vi "Lab 2 Part B.vi"() -> ()   [LabVIEW 2020]
uses:
  <vilib>/MakerHub/LINX/Public/Utilities/Open Serial.vi
  <vilib>/addons/control/pid/pid.llb/PID (DBL).vi
  <vilib>/MakerHub/LINX/LMH-LINX.lvlib
  <vilib>/addons/control/pid/NI_PID_pid.lvlib
panel:
  in  "Amplitude":dbl=0.5
  in  "Frequency":dbl=0.01
  in  "Offset":dbl=1.5
  in  "PWM Channel":u8=10
  in  "AI1 and AI2 Channels":u8[](array[numeric])
  in  "Hall Channel":u8
  in  "Stop Button":bool
  out "Voltage":dbl
  in  "PID gains":T1={"proportional gain (Kc)"=5.0, "integral time (Ti, min)"=0.003, "derivative time (Td, min)"=0.01} {"derivative time (Td, min)" format="%.6f"; "integral time (Ti, min)" format="%.6f"; "proportional gain (Kc)" format="%.3f"}
  out "Output Chart":dynamicdata(graph)
  in  "output range":cluster{"output high":dbl, "output low":dbl}={"output high"=100.0, "output low"=-100.0} {"output low" format="%.2f"; "output high" format="%.2f"}
  out "Duty Cycle":dbl
  in  "Serial Port":refnum<visa-resource-name>="N/A"
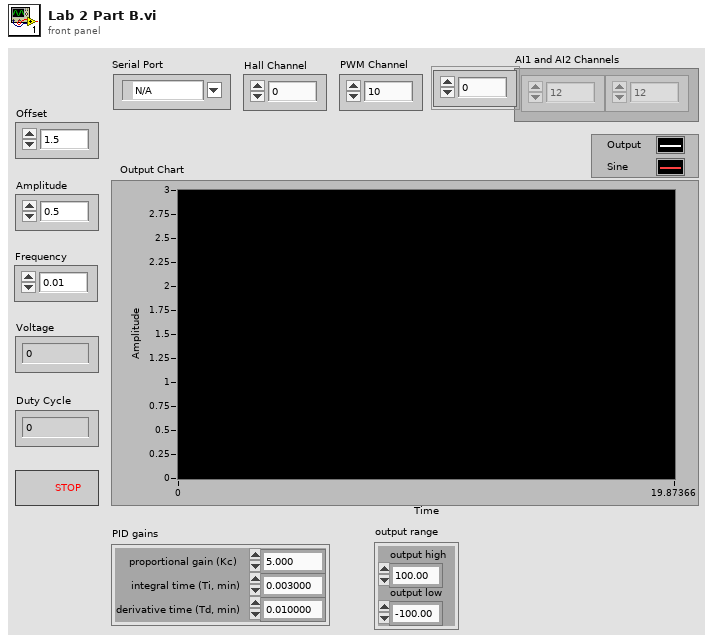
[diagram p1: front panel]
types:
  T1 = cluster{"proportional gain (Kc)":dbl, "integral time (Ti, min)":dbl, "derivative time (Td, min)":dbl}
  T2 = typedef "LMH-LINX.lvlib/LINX Ref.ctl" = cluster{"IO":T3, "Interface":T4, "LINX Device Config":T5}
  T3 = typedef "LMH-LINX.lvlib/Platform.ctl" = enum16{"Remote", "Local"}
  T4 = typedef "LMH-LINX.lvlib/Interface.ctl" = enum16{"Serial", "TCP"}
  T5 = typedef "LMH-LINX.lvlib/Device.lvlib/LINX Device Config.ctl" = cluster{"Interface":T4, "COM Port":refnum<visa-resource-name>, "TCP Configuration":T6, "Device Family":u8, "Device ID":u8, "Device Name":string, "TCP Ref":refnum<k5>, "Channels":T7}
  T6 = typedef "LMH-LINX.lvlib/Device.lvlib/TCP Config.ctl" = cluster{"IP Address":string, "Port":u16}
  T7 = typedef "LMH-LINX.lvlib/Channels.ctl" = cluster{"DI":u8[], "DO":u8[], "AI":u8[], "AO":u8[], "PWM":u8[], "QE":u8[], "UART":u8[], "I2C 2":u8[], "SPI":u8[], "CAN":u8[], "Servo":u8[], "AI Ref (V)":dbl, "AI Resolution (Bits)":u8, "AO Ref (V)":dbl, "AO Resolution (Bits)":u8}
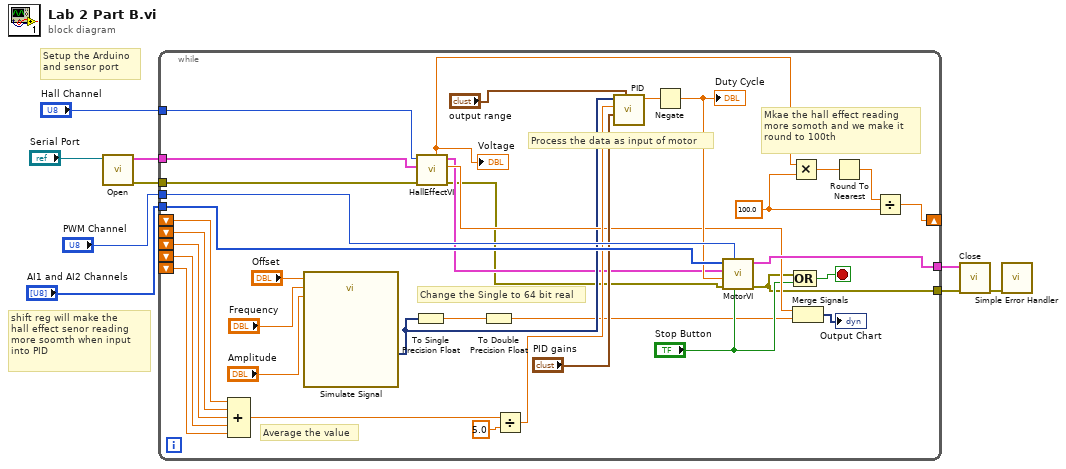
[diagram p0: block diagram]
diagram:
  # "shift reg will make the\nhall effect senor reading\nmore soomth when input \ninto PID"
  # "Setup the Arduino\nand sensor port"
  n1 = call-poly <vilib>:"Open.vi"("Serial Port"="Serial Port") -> ("Error Out"=w4:errorcluster, "LINX Resource"=w5:T2)  [unwired: 8 in, 1 out]
  n2 = while {
    tunnel: "Hall Channel" -> [w45]
    tunnel: "AI1 and AI2 Channels" -> [w44]
    tunnel: "PWM Channel" -> [w43]
    tunnel: w5 -> [w42]
    tunnel: w4 -> [w38]
    tunnel: [w39] -> w3
    tunnel: [w10] -> w2
    shift-right: [w23] -> _
    shift-left: _ -> [w36]
    shift-left: _ -> [w35]
    shift-left: _ -> [w34]
    shift-left: _ -> [w33]
    shift-left: _ -> [w29]
    stop <- w37 stop-if-true
    w24 = 100.0 ("y")
    # "Change the Single to 64 bit real"
    # "Average the value"
    # "Process the data as input of motor"
    # "Mkae the hall effect reading\nmore somoth and we make it\nround to 100th"
    n3 = Compound Arithmetic op=ADD(w36, w35, w34, w33, w29) -> (w32:dbl)
    n4 = call "Simulate Signal"("Offset"="Offset", "Frequency"="Frequency", "Amplitude"="Amplitude") -> ("Sine"=w16:dynamicdata)  [unwired: 11 in, 1 out]
    n5 = To Single Precision Float(number=w16) -> (single precision float=w13:sgl)
    n6 = call "HallEffectVI.vi"("error in (no error)"=w38, "LINX Resource in"=w42, "Analog Channel"=w45) -> ("error out"=w11:errorcluster, "Waveform Chart"=w22:dbl, "LINX Resource out"=w12:T2, "Voltage"=w27:dbl)  [unwired: 5 in]
    "Voltage" <- w27
    n7 = To Double Precision Float(number=w13) -> (double precision float=w14:dbl)
    n8 = Divide(x=w32, y=5.0) -> (x/y=w28:dbl)
    n9 = call-poly <vilib>:"PID.vi"("output range"="output range", "PID gains"="PID gains", "process variable"=w28, "setpoint"=w16) -> ("output"=w17:dbl)  [unwired: 6 in, 1 out]
    n10 = Negate(x=w17) -> (-x=w30:dbl)
    "Duty Cycle" <- w30
    n11 = call "MotorVI.vi"("stop"="Stop Button", "PWM Channel"=w43, "error in (no error)"=w11, "Duty Cycle (-100 to +100)"=w30, "LINX Resource in"=w12, "AI1 and AI2 Channels"=w44) -> ("error out"=w10:errorcluster, "LINX Resource out"=w39:T2)  [unwired: 3 in, 1 out]
    n12 = Multiply(x=w27, y=w24) -> (x*y=w26:dbl)
    n13 = Merge Signals(w22, w14) -> (→"Output Chart":dynamicdata)
    n14 = Compound Arithmetic op=OR(w10, "Stop Button") -> (w37:bool)
    n15 = Round To Nearest(number=w26) -> (nearest integer value=w25:dbl)
    n16 = Divide(x=w25, y=w24) -> (x/y=w23:dbl)
  }
  n17 = call <vilib>:"Close.vi"("Error In"=w2, "LINX Resource"=w3) -> ("Error Out"=w1:errorcluster)  [unwired: 9 in]
  n18 = call <vilib>:"Simple Error Handler.vi"("error in (no error)"=w1) -> ()  [unwired: 4 in, 5 out]
